vi "Msg - Queue Manager Mode_2.vi"(0 "Mode":T1, 5 "Module Name":string, 11 "error in (no error)":errorcluster) -> (4 ">>ThisModule":refnum<queue>, 6 ">>Controller":refnum<queue>, 15 "error out":errorcluster)   [LabVIEW 2017, in "Error Handler - Logger.lvlib"]
doc: "Template used to create VIs that belong to this Module."
uses:
  Error Handler - Logger.lvlib
  Controls/Message - Queue Manager Mode.ctl
  Controls/Module - Data.ctl
  Modules.ctl
  Controls/Module - States.ctl
  Controls/Timing - Data.ctl
  Controls/Process - Element.ctl
  Controls/Process.ctl
  Controls/Process - Status.ctl
  Controls/Current Error Details.ctl
  Controls/Error Types.ctl
  Controls/Message.ctl
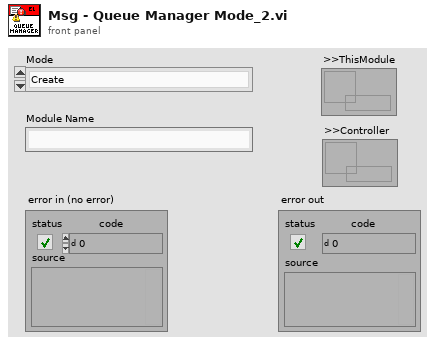
[diagram p1: front panel]
types:
  T1 = typedef "Error Handler - Logger.lvlib/Message - Queue Manager Mode.ctl" = enum16{"Create", "Get", "Destroy"}
  T2 = typedef "Error Handler - Logger.lvlib/Module - Data.ctl" = cluster{"This Module":T3, "Current State":T4, "Timing Data":T5, "Processes":T6[], "Current Error":T9}
  T3 = typedef "Error Handler - Logger.lvlib/Modules.ctl" = enum16{"Controller", "Error Handler - Logger"}
  T4 = typedef "Error Handler - Logger.lvlib/Module - States.ctl" = enum16{"Initialize", "Event ", "Send data", "FP Element: Update", "FP Element: Disable/Enable", "Timer: Setup", "Terminate", "--------Template----------", "Process Error", "Log ", "Log Error"}
  T5 = typedef "Error Handler - Logger.lvlib/Timing - Data.ctl" = cluster{"Elapsed Time":dbl, "Time Target":dbl, "Time Stamp":timestamp, "Paused?":bool, "Reached?":bool}
  T6 = typedef "Error Handler - Logger.lvlib/Process - Element.ctl" = cluster{"Process":T7, "Status":T8, "Data":variant}
  T7 = typedef "Error Handler - Logger.lvlib/Process.ctl" = enum16{""}
  T8 = typedef "Error Handler - Logger.lvlib/Process - Status.ctl" = enum16{"Uninitialized", "Busy"}
  T9 = typedef "Error Handler - Logger.lvlib/Current Error Details.ctl" = cluster{"Current Error Type":T10, "Error":errorcluster}
  T10 = typedef "Error Handler - Logger.lvlib/Error Types.ctl" = enum16{""}
  T11 = typedef "Error Handler - Logger.lvlib/Message.ctl" = cluster{"State":T4, "Data":variant, "Originating Module":T3}
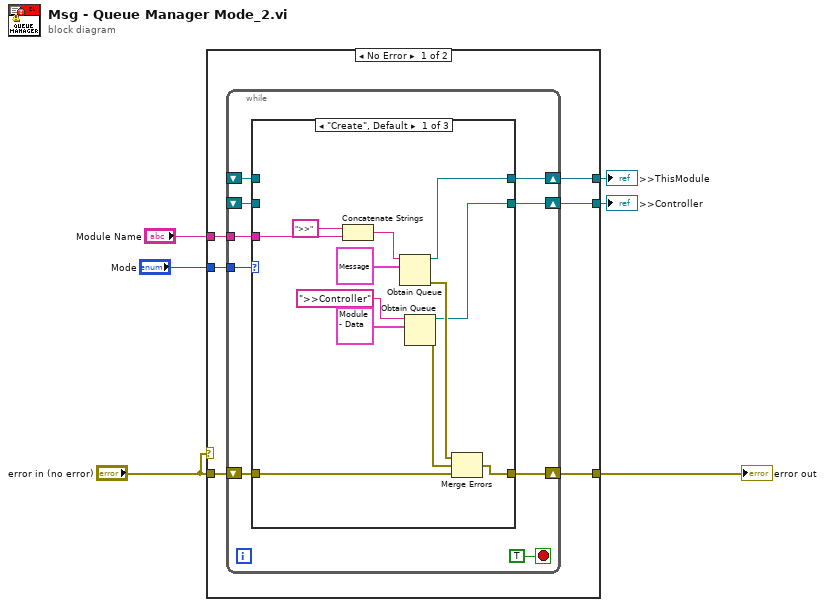
[diagram p0: block diagram]
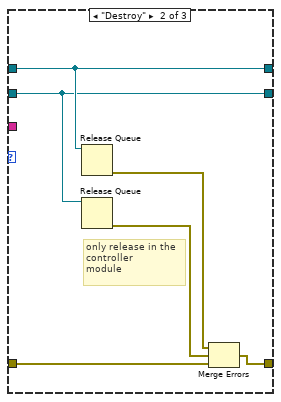
[diagram p2: hidden frame]
diagram:
  n1 = case shown="No Error" "error in (no error)" {
    tunnel: [w12 _] -> w1
    tunnel: [w11 w43] -> w6
    tunnel: "error in (no error)" -> [w10 w43]
    tunnel: [w9 _] -> w3
    tunnel: "Mode" -> [w8 _]
    tunnel: "Module Name" -> [w7 _]
    frame No Error {
      n2 = while {
        shift-right: [w21] -> w12
        shift-left: _ -> [w20]
        shift-right: [w19] -> w11
        shift-left: w10 -> [w18]
        shift-right: [w15] -> w9
        shift-left: _ -> [w16]
        tunnel: w8 -> [w14]
        tunnel: w7 -> [w13]
        stop <- TRUE stop-if-true
        n3 = case shown="\"Create\", Default" w14 {
          tunnel: [w29 w37 w42] -> w21
          tunnel: w20 -> [_ w37 w42]
          tunnel: [w32 w38 w41] -> w19
          tunnel: w18 -> [w33 w39 w41]
          tunnel: [w28 w36 w40] -> w15
          tunnel: w16 -> [_ w36 w40]
          tunnel: w13 -> [w24 _ _]
          frame "Create", Default {
            n4 = Concatenate Strings(">>" ("string"), w24) -> (w23:string)
            n5 = Obtain Queue(name (unnamed)=w23, element data type=T11 {"State"=enum."Initialize", "Data"=variant, "Originating Module"=enum."Controller"} ("Message")) -> (queue out=w29:refnum<queue>, error out=w31:errorcluster)  [unwired: 3 in, 1 out]
            n6 = Obtain Queue(name (unnamed)=">>Controller", element data type=T2 {"This Module"=enum."Controller", "Current State"=enum."Initialize", "Timing Data"={"Elapsed Time"=0.0, "Time Target"=0.0, "Time Stamp"=timestamp(0 s since 1904-01-01), "Paused?"=FALSE, "Reached?"=FALSE}, "Processes"=[], "Current Error"={"Current Error Type"=enum."", "Error"={"status"=FALSE, "code"=0, "source"=""}}} ("Module Data")) -> (queue out=w28:refnum<queue>, error out=w30:errorcluster)  [unwired: 3 in, 1 out]
            n7 = Merge Errors(w31, w30, w33) -> (w32:errorcluster)
          }
          frame "Destroy" {
            # "only release in the \ncontroller \nmodule"
            n8 = Release Queue(queue=w37) -> (error out=w35:errorcluster)  [unwired: 2 in, 2 out]
            n9 = Release Queue(queue=w36) -> (error out=w34:errorcluster)  [unwired: 2 in, 2 out]
            n10 = Merge Errors(w35, w34, w39) -> (w38:errorcluster)
          }
          frame "Get" {
          }
        }
      }
    }
    frame Error {
    }
  }
  "error out" <- w6
  ">>Controller" <- w3
  ">>ThisModule" <- w1
